vi "Profile_minus_Mean.vi"() -> (0 "New Values In":string[][](array[string])=[["Test data5"]], 1 "New Chs In":string[](array[string])=["30-10-03:New:Channel new5"])   [LabVIEW 2020]
uses:
  Results_plotter_Global.vi
  <vilib>/Analysis/NI_AALBase.lvlib
  Data plotting/subVIs/Plot_Values_Global.vi
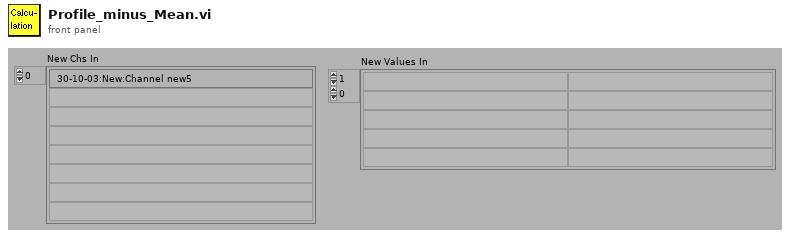
[diagram p1: front panel]
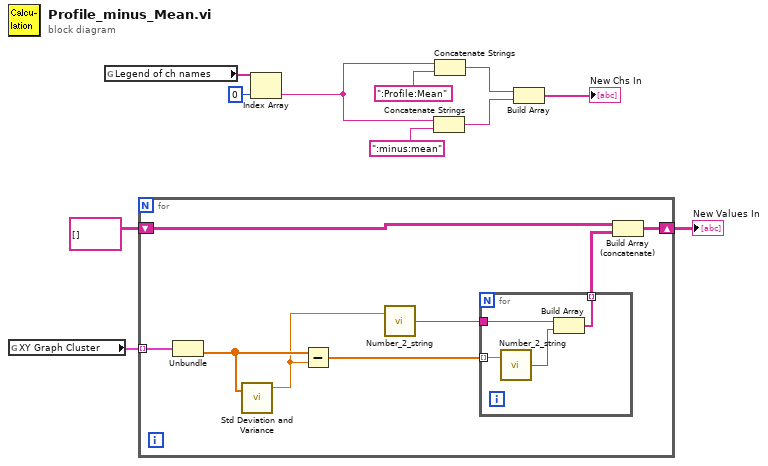
[diagram p0: block diagram]
diagram:
  n1 = global read "Plot_Values_Global.vi" "XY Graph Cluster"() -> (w1:cluster{dbl[], dbl[]}[])
  n2 = global read "Results_plotter_Global.vi" "Legend of ch names"() -> (w8:string[])
  n3 = for {
    tunnel: w1 -> [w19] mode=indexing
    shift-right: [w15] -> w5
    shift-left: string[][] [] -> [w17]
    n4 = Unbundle(w19) -> (w18:dbl[])  [unwired: 1 out]
    n5 = call <vilib>:"Std Deviation and Variance.vi"("X"=w18) -> ("mean"=w14:dbl)  [unwired: 1 in, 2 out]
    n6 = Subtract(x=w18, y=w14) -> (x-y=w12:dbl[])
    n7 = call "Number_2_string.vi"("number"=w14) -> ("String"=w13:string)  [unwired: 1 in]
    n8 = for {
      tunnel: w12 -> [w23] mode=indexing
      tunnel: [w21] -> w16 mode=indexing
      tunnel: w13 -> [w20]
      n9 = call "Number_2_string.vi"("number"=w23) -> ("String"=w22:string)  [unwired: 1 in]
      n10 = Build Array(w20, w22) -> (w21:string[])
    }
    n11 = Build Array (concatenate)(w17, w16) -> (w15:string[][])
  }
  "New Values In" <- w5
  n12 = Index Array(array=w8, index=0) -> (element=w3:string)
  n13 = Concatenate Strings(w3, ":minus:mean" ("string")) -> (w6:string)
  n14 = Concatenate Strings(w3, ":Profile:Mean" ("string")) -> (w2:string)
  n15 = Build Array(w2, w6) -> (→"New Chs In":string[])
